vi "Thermoflex Checksum.vi"(10 "Pad":bool=TRUE, 11 "String in":string) -> (2 "Checksum String":string, 3 "result string":string)   [LabVIEW 2021, in "SMC Protection.lvclass"]
uses:
  SMC Protection.lvclass
  SMC Protection.lvclass/SMC Protection.ctl
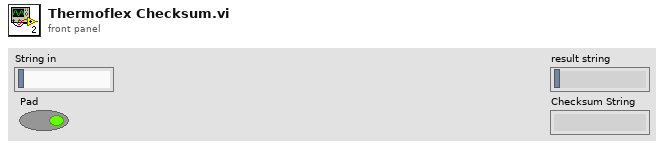
[diagram p1: front panel]
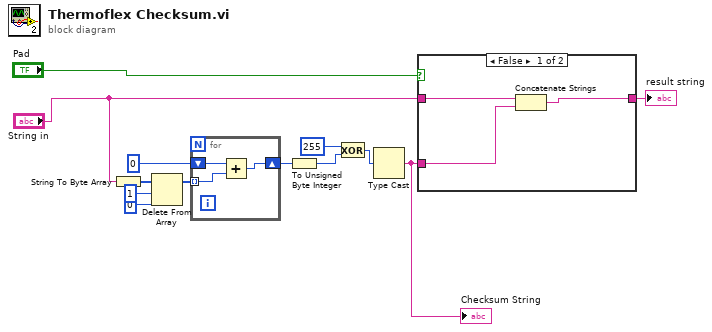
[diagram p0: block diagram]
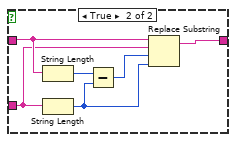
[diagram p2: hidden frame]
diagram:
  n1 = String To Byte Array(string="String in") -> (unsigned byte array=w13:u8[])
  n2 = Delete From Array(array=w13, length=1, index=0) -> (array with subset deleted=w6:u8[])  [unwired: 1 out]
  n3 = for {
    tunnel: w6 -> [w16] mode=indexing
    shift-right: [w14] -> w11
    shift-left: u64 0 -> [w15]
    n4 = Add(x=w15, y=w16) -> (x+y=w14:u64)
  }
  n5 = To Unsigned Byte Integer(number=w11) -> (unsigned 8bit integer=w8:u8)
  n6 = Exclusive Or(1:w8, 2:u8 255 ("x")) -> (0:w7:u8)
  n7 = Type Cast(x=w7) -> (*(type *) &x=w10:string)  [unwired: 1 in]
  "Checksum String" <- w10
  n8 = case shown="False" "Pad" {
    tunnel: w10 -> [w19 w20]
    tunnel: "String in" -> [w18 w24]
    tunnel: [w17 w25] -> w1
    frame False {
      n9 = Concatenate Strings(w18, w19) -> (w17:string)
    }
    frame True {
      n10 = String Length(string=w24) -> (length=w23:i32)
      n11 = String Length(string=w20) -> (length=w22:i32)
      n12 = Subtract(x=w23, y=w22) -> (x-y=w21:i32)
      n13 = Replace Substring(2:w22, 3:w21, 4:w20, 5:w24) -> (1:w25:string)  [unwired: 1 out]
    }
  }
  "result string" <- w1
